vi "DeCoF VISA resources with filter.vi"(4 "error in (no error)":errorcluster, 5 "apply filter":bool, 6 "filter expression":string="COM") -> (0 "error out":errorcluster, 2 "Array":T1(array[cluster]))   [LabVIEW 2013]
doc: "This VI returns a list of the RS232 ports available on the PC."
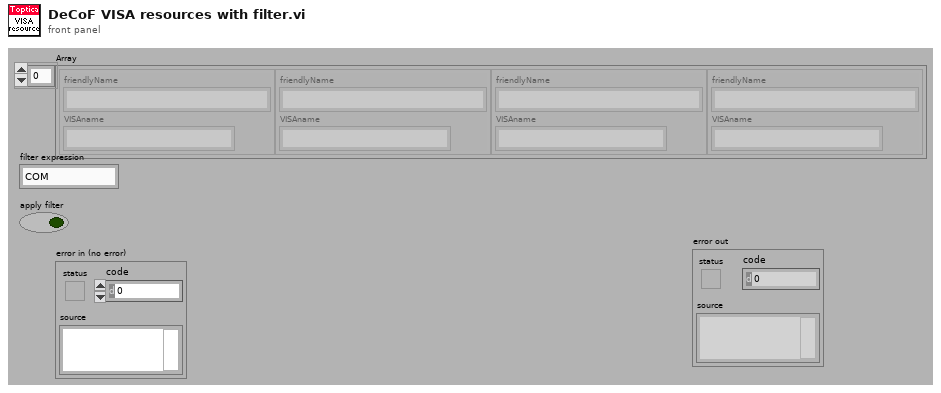
[diagram p1: front panel]
types:
  T1 = cluster{"friendlyName":string, "VISAname":string}[]
  T2 = cluster{"Intf Inst Name":string, "VISAname":string}[]
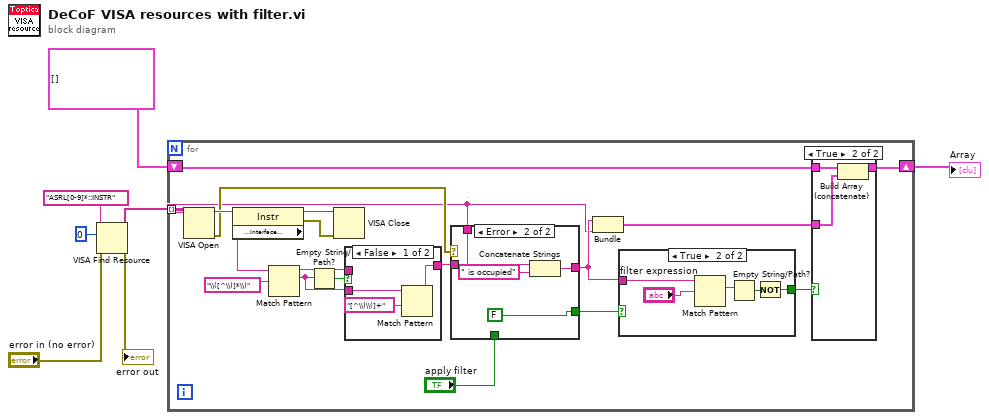
[diagram p0: block diagram]
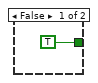
[diagram p3: hidden frame]
diagram:
  n1 = VISA Find Resource(8:"error in (no error)", 10:u32 0 ("search mode (0)"), 11:"ASRL[0-9]*::INSTR" ("expression (\"?*\")")) -> (0:→"error out":errorcluster, 3:w6:string[])  [unwired: 1 out]
  n2 = for {
    tunnel: w6 -> [w8] mode=indexing
    shift-right: [w14] -> w4
    shift-left: T1 [] -> [w13]
    n3 = VISA Open(VISA resource name=w8) -> (VISA resource name=w25:refnum<visa-resource-name>, error out=w18:errorcluster)  [unwired: 4 in]
    n4 = property class="Instr"(reference=w25) -> (reference out=w24:refnum<visa-resource-name>, error out=w23:errorcluster, "Interface Information:Interface Description"=w16:string)  [unwired: 1 in]
    n5 = Match Pattern(string=w16, regular expression="\\([^\\)]*\\)") -> (before substring=w20:string, match substring=w19:string)  [unwired: 1 in, 2 out]
    n6 = Empty String/Path?(string/path=w19) -> (empty?=w21:bool)
    n7 = VISA Close(VISA resource name=w24, error in (no error)=w23) -> ()  [unwired: 1 out]
    n8 = case shown="False" w21 {
      tunnel: w20 -> [_ w45]
      tunnel: w19 -> [w43 _]
      tunnel: [w42 w45] -> w17
      frame False {
        n9 = Match Pattern(string=w43, regular expression="[^\\)\\(]+") -> (match substring=w42:string)  [unwired: 1 in, 3 out]
      }
      frame True {
      }
    }
    n10 = case shown="Error" w18 {
      tunnel: w17 -> [w37 _]
      tunnel: [w37 w40] -> w15
      tunnel: [w36 FALSE] -> w9
      tunnel: "apply filter" -> [w36 _]
      tunnel: w8 -> [_ w39]
      frame No Error {
      }
      frame Error {
        n11 = Concatenate Strings(w39, " is occupied" ("string")) -> (w40:string)
      }
    }
    n12 = Bundle("Intf Inst Name"=w15, w8) -> (w12:cluster{"Intf Inst Name":string, string})  [unwired: 1 in]
    n13 = case shown="True" w9 {
      tunnel: w15 -> [_ w35]
      tunnel: [TRUE w31] -> w11
      frame False {
      }
      frame True {
        n14 = Match Pattern(string=w35, regular expression="filter expression") -> (match substring=w33:string)  [unwired: 1 in, 3 out]
        n15 = Empty String/Path?(string/path=w33) -> (empty?=w32:bool)
        n16 = Not(x=w32) -> (.not. x?=w31:bool)
      }
    }
    n17 = case shown="True" w11 {
      tunnel: [w26 w29] -> w14
      tunnel: w13 -> [w26 w28]
      tunnel: w12 -> [_ w27]
      frame False {
      }
      frame True {
        n18 = Build Array (concatenate)(w28, w27) -> (w29:T2)
      }
    }
  }
  "Array" <- w4
